vi "Parse Response.vi"(8 "error in (no error)":errorcluster, 10 "header":string, 11 "body in":string) -> (0 "error out":errorcluster, 2 "id":dbl, 3 "body out":string, 4 "error data":string[](array[string]))   [LabVIEW 2017, in "Random JSON API.lvlib"]
uses:
  Random JSON API.lvlib
  <vilib>/regexp/Match Regular Expression.xnode
  <vilib>/ErrorRing/Error Ring.xnode
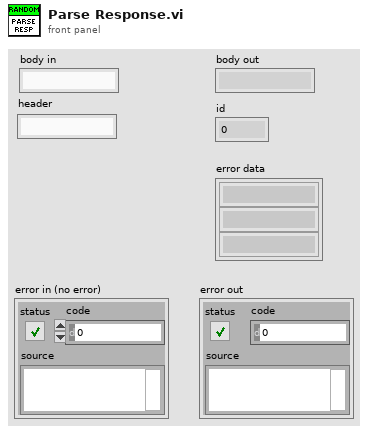
[diagram p1: front panel]
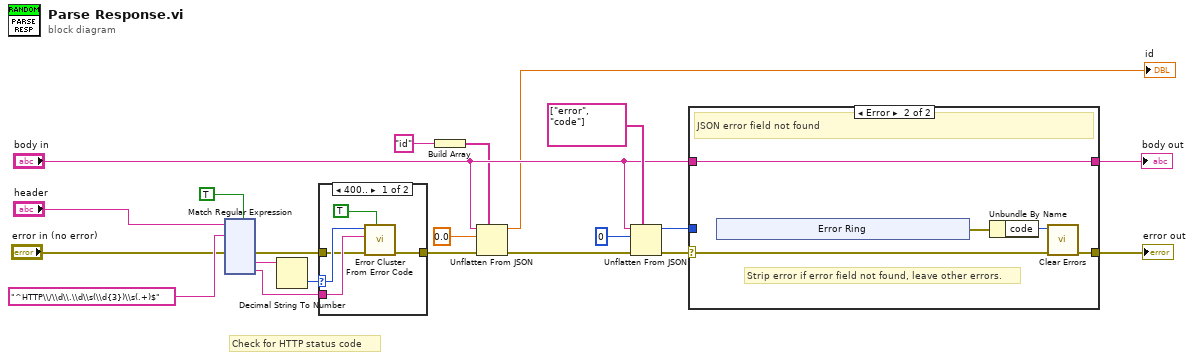
[diagram p0: block diagram]
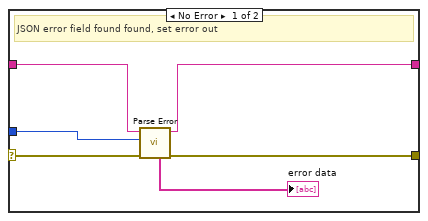
[diagram p3: hidden frame]
diagram:
  # "Check for HTTP status code"
  n1 = xnode "Match Regular Expression"("input string"="header", "regular expression"="^HTTP\\/\\d\\.\\d\\s(\\d{3})\\s(.+)$", "error in"="error in (no error)", "multiline? (F)"=TRUE ("ignore case? (F)")) -> ("error out"=w16:errorcluster, "submatch 1"=w21:string, "submatch 2"=w17:string)  [unwired: 2 in, 4 out]
  n2 = Decimal String To Number(string=w21) -> (number=w18:i32)  [unwired: 2 in, 1 out]
  n3 = case shown="400.." w18 {
    selector: w18 -> [w26 _]
    tunnel: [w23 w27] -> w7
    tunnel: w17 -> [w25 _]
    tunnel: w16 -> [w24 w27]
    frame 400.. {
      n4 = call <vilib>:"Error Cluster From Error Code.vi"("show call chain? (False)"=TRUE, "error in (no error)"=w24, "error message (\"\")"=w25, "error code (0)"=w26) -> ("error out"=w23:errorcluster)  [unwired: 5 in]
    }
    frame Default {
    }
  }
  n5 = Build Array("id") -> (w1:string[])
  n6 = Unflatten From JSON(path=w1, JSON string="body in", type and defaults=0.0, error in (no error)=w7) -> (value=→"id":dbl, error out=w6:errorcluster)  [unwired: 3 in]
  n7 = Unflatten From JSON(path=string[] ["error", "code"], JSON string="body in", type and defaults=0, error in (no error)=w6) -> (value=w9:i32, error out=w12:errorcluster)  [unwired: 3 in]
  n8 = case shown="Error" w12 {
    selector: w12 -> [w30 w35]
    tunnel: [w32 w34] -> w13
    tunnel: w9 -> [w33 _]
    tunnel: "body in" -> [w31 w38]
    tunnel: [w29 w38] -> w8
    frame No Error {
      # "JSON error field found found, set error out"
      n9 = call "Parse Error.vi"("error in (no error)"=w30, "error code"=w33, "body in"=w31) -> ("error out"=w32:errorcluster, "body out"=w29:string, "error data"=→"error data":string[])  [unwired: 6 in]
    }
    frame Error {
      # "Strip error if error field not found, leave other errors."
      # "JSON error field not found"
      n10 = xnode "Error Ring"() -> ("error out"=w37:errorcluster)
      n11 = Unbundle By Name(w37) -> ("code"=w36:i32)
      n12 = call <vilib>:"Clear Errors.vi"("error in (no error)"=w35, "specific error code to clear (0: all)"=w36) -> ("error out"=w34:errorcluster)  [unwired: 4 in, 1 out]
    }
  }
  "error out" <- w13
  "body out" <- w8
